vi "计算结果到报表.vi"(0 "步响应计算参数":T1, 1 "计算参数":T2, 2 "试验模式":string, 3 "试验报表路径":path) -> ()   [LabVIEW 2013]
doc: "该函数将计算所得的参数写入到试验报表的文本文档里。"
uses:
  <vilib>/Utility/config.llb/Write Key (String).vi
  <vilib>/Utility/config.llb/Write Key (Double).vi
  <vilib>/Utility/config.llb/NI_LVConfig.lvlib
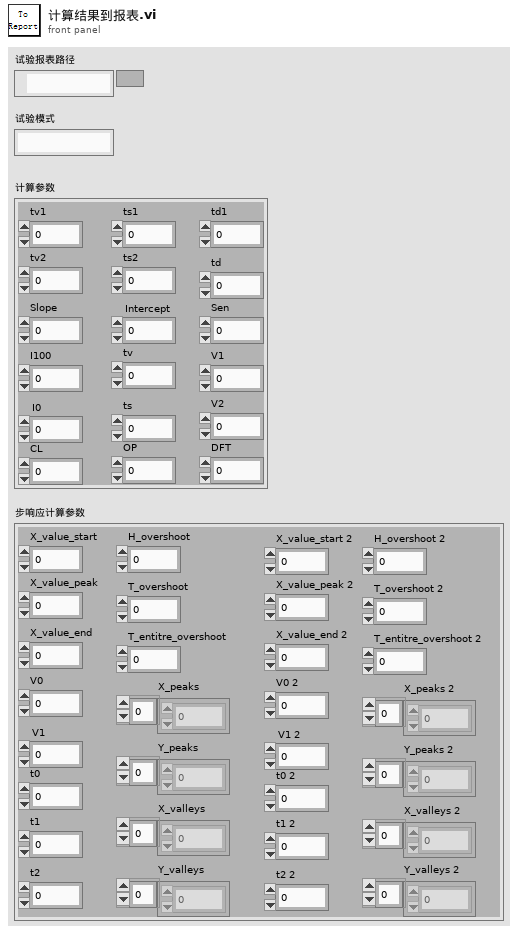
[diagram p1: front panel]
types:
  T1 = cluster{"X_value_start":dbl, "X_value_peak":dbl, "t1":dbl, "X_value_end":dbl, "V0":dbl, "V1":dbl, "t0":dbl, "X_peaks":dbl[], "X_valleys":dbl[], "Y_peaks":dbl[], "Y_valleys":dbl[], "t2":dbl, "H_overshoot":dbl, "T_overshoot":dbl, "T_entitre_overshoot":dbl, "X_value_start 2":dbl, "X_value_peak 2":dbl, "t1 2":dbl, "X_value_end 2":dbl, "V0 2":dbl, "V1 2":dbl, "t0 2":dbl, "X_peaks 2":dbl[], "X_valleys 2":dbl[], "Y_peaks 2":dbl[], "t2 2":dbl, "H_overshoot 2":dbl, "T_overshoot 2":dbl, "T_entitre_overshoot 2":dbl, "Y_valleys 2":dbl[]}
  T2 = cluster{"tv1":dbl, "tv2":dbl, "tv":dbl, "ts1":dbl, "ts2":dbl, "ts":dbl, "td1":dbl, "td":dbl, "Slope":dbl, "Intercept":dbl, "I100":dbl, "I0":dbl, "Sen":dbl, "V1":dbl, "V2":dbl, "CL":dbl, "OP":dbl, "DFT":dbl}
  T3 = typedef "NI_LVConfig.lvlib/Config Data RefNum.ctl" = refnum<k1>
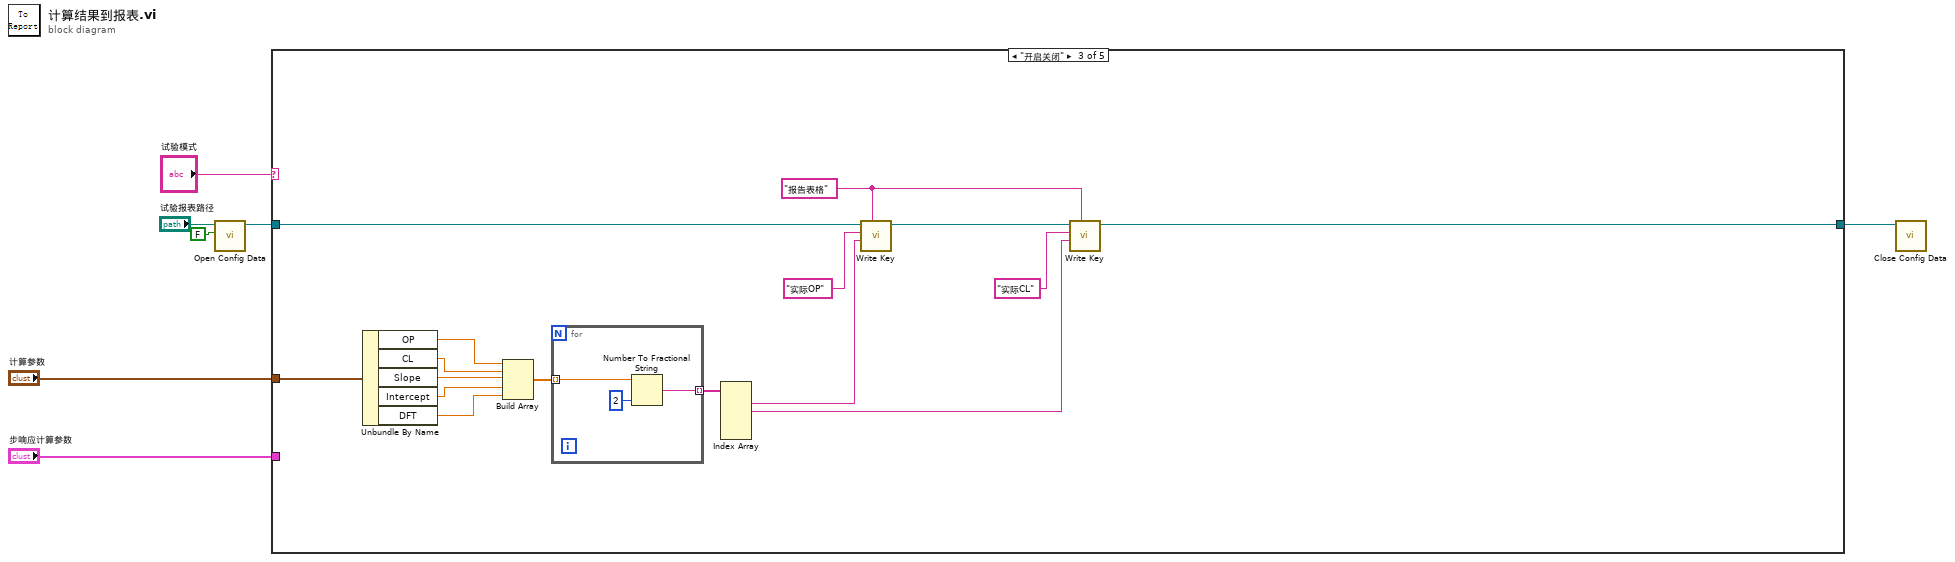
[diagram p0: block diagram]
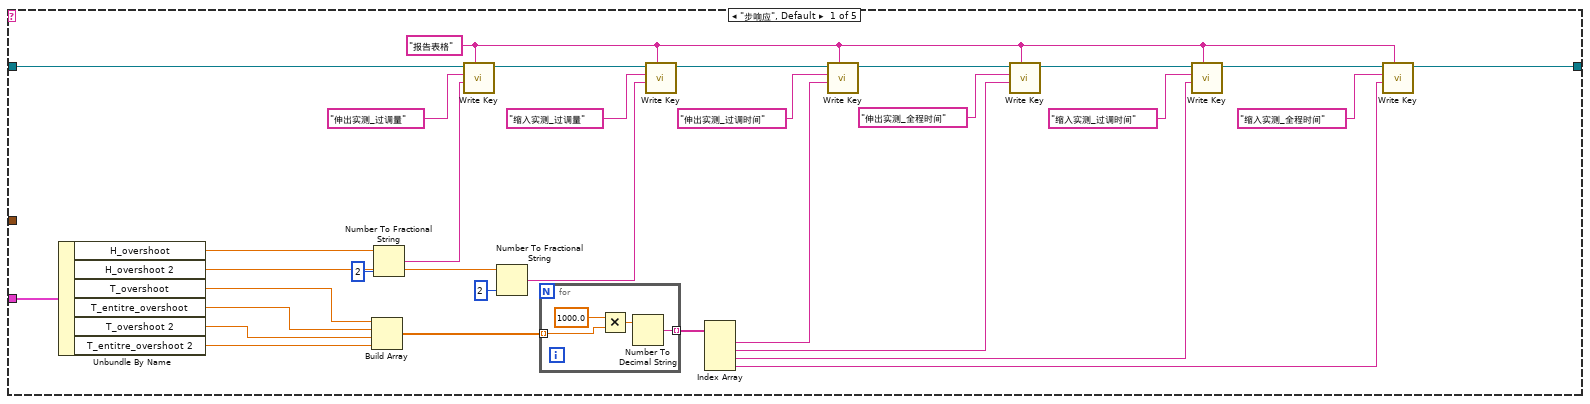
[diagram p2: hidden frame]
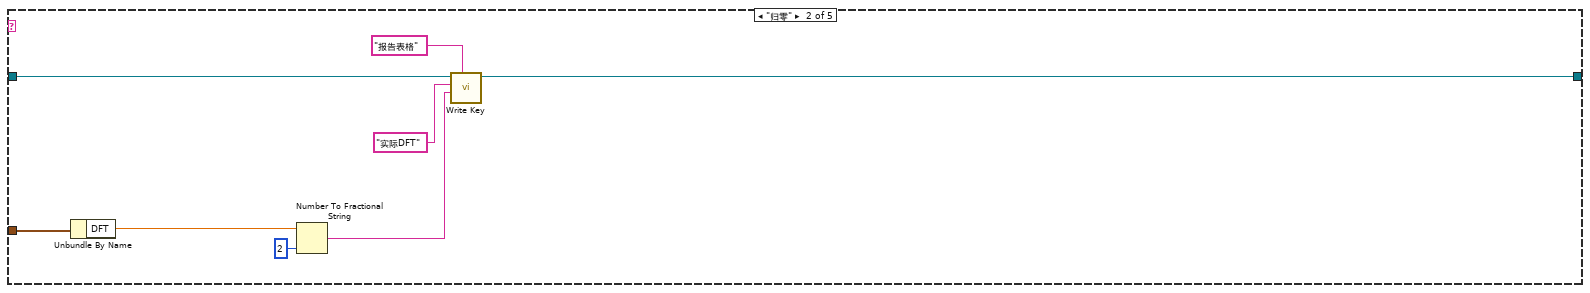
[diagram p3: hidden frame]
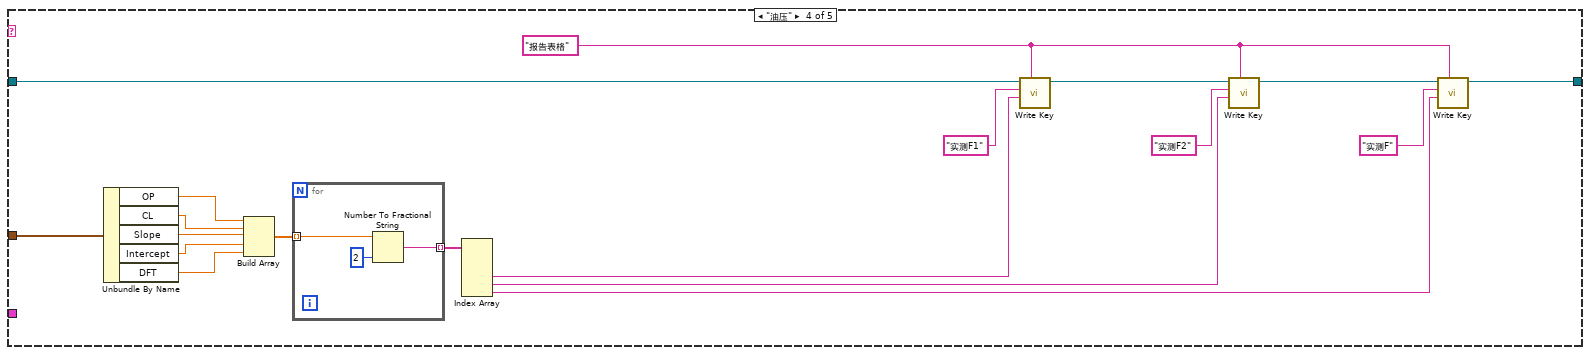
[diagram p4: hidden frame]
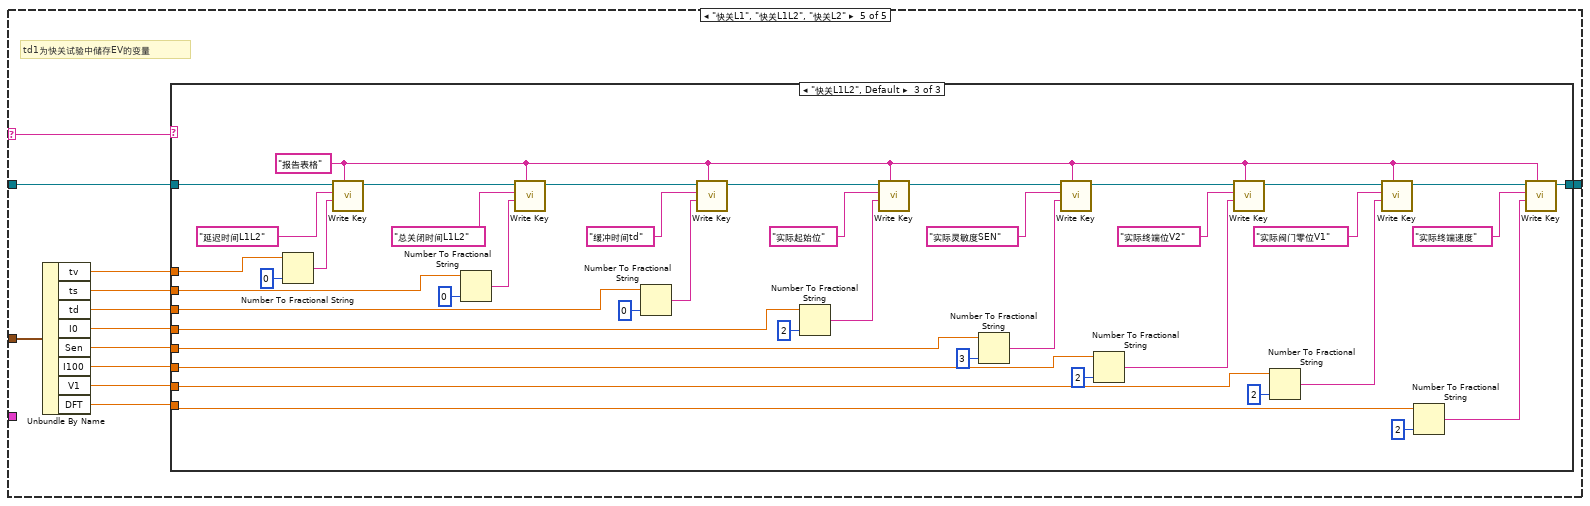
[diagram p5: hidden frame]
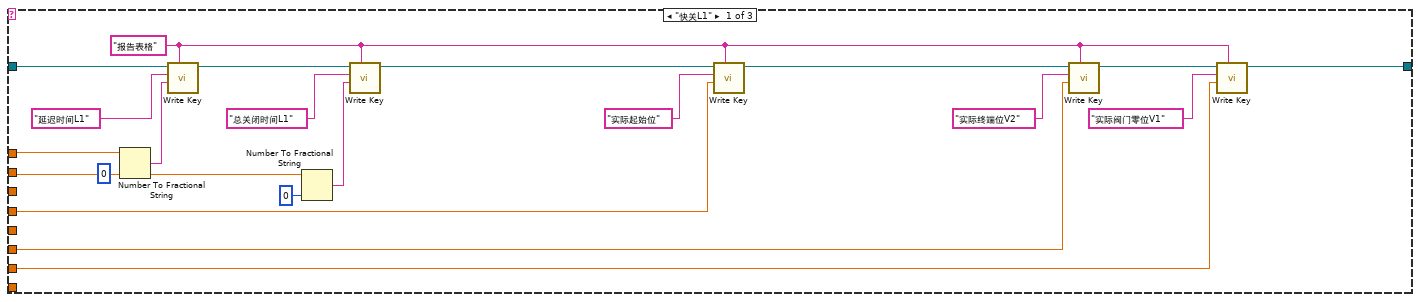
[diagram p6: hidden frame]
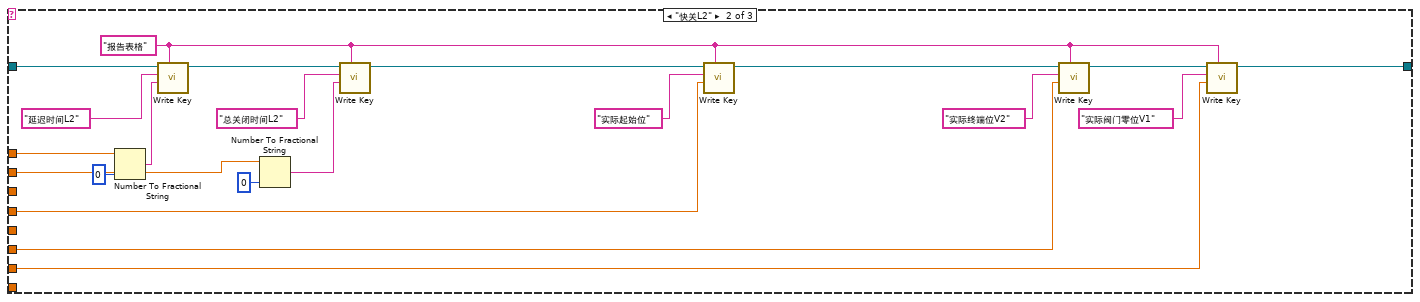
[diagram p7: hidden frame]
diagram:
  n1 = call <vilib>:"Open Config Data.vi"("create file if necessary (T)"=FALSE, "configuration file path"="试验报表路径") -> ("refnum"=w4:T3)  [unwired: 7 in, 2 out]
  n2 = case shown="\"开启关闭\"" "试验模式" {
    selector: "试验模式" -> [_ _ _ _ w103]
    tunnel: "计算参数" -> [_ w50 w66 w71 w102]
    tunnel: w4 -> [w29 w47 w62 w70 w101]
    tunnel: [w24 w46 w51 w72 w100] -> w3
    tunnel: "步响应计算参数" -> [w28 _ _ _ _]
    frame "步响应", Default {
      w26 = "报告表格"
      n3 = Unbundle By Name(w28) -> ("H_overshoot"=w12:dbl, "H_overshoot 2"=w9:dbl, "T_overshoot"=w20:dbl, "T_entitre_overshoot"=w21:dbl, "T_overshoot 2"=w18:dbl, "T_entitre_overshoot 2"=w22:dbl)
      n4 = Build Array(w20, w21, w18, w22) -> (w23:dbl[])
      n5 = Number To Fractional String(number=w12, precision (6)=i16 2) -> (F-format string=w11:string)  [unwired: 2 in]
      n6 = call-poly <vilib>:"Write Key.vi"("section"=w26, "value"=w11, "key"="伸出实测_过调量", "refnum"=w29) -> ("refnum out"=w33:T3)  [unwired: 5 in, 2 out]
      n7 = Number To Fractional String(number=w9, precision (6)=i16 2) -> (F-format string=w8:string)  [unwired: 2 in]
      n8 = for {
        tunnel: w23 -> [w41] mode=indexing
        tunnel: [w39] -> w19 mode=indexing
        n9 = Multiply(x=1000.0, y=w41) -> (x*y=w40:dbl)
        n10 = Number To Decimal String(number=w40) -> (decimal integer string=w39:string)  [unwired: 1 in]
      }
      n11 = call-poly <vilib>:"Write Key.vi"("section"=w26, "value"=w8, "key"="缩入实测_过调量", "refnum"=w33) -> ("refnum out"=w32:T3)  [unwired: 5 in, 2 out]
      n12 = Index Array(array=w19) -> (element #1=w17:string, element #2=w16:string, element #3=w15:string, element #4=w14:string)  [unwired: 4 in]
      n13 = call-poly <vilib>:"Write Key.vi"("section"=w26, "value"=w17, "key"="伸出实测_过调时间", "refnum"=w32) -> ("refnum out"=w31:T3)  [unwired: 5 in, 2 out]
      n14 = call-poly <vilib>:"Write Key.vi"("section"=w26, "value"=w16, "key"="伸出实测_全程时间", "refnum"=w31) -> ("refnum out"=w30:T3)  [unwired: 5 in, 2 out]
      n15 = call-poly <vilib>:"Write Key.vi"("section"=w26, "value"=w15, "key"="缩入实测_过调时间", "refnum"=w30) -> ("refnum out"=w25:T3)  [unwired: 5 in, 2 out]
      n16 = call-poly <vilib>:"Write Key.vi"("section"=w26, "value"=w14, "key"="缩入实测_全程时间", "refnum"=w25) -> ("refnum out"=w24:T3)  [unwired: 5 in, 2 out]
    }
    frame "归零" {
      n17 = Unbundle By Name(w50) -> ("DFT"=w45:dbl)
      n18 = Number To Fractional String(number=w45, precision (6)=i16 2) -> (F-format string=w44:string)  [unwired: 2 in]
      n19 = call-poly <vilib>:"Write Key.vi"("section"="报告表格", "value"=w44, "key"="实际DFT", "refnum"=w47) -> ("refnum out"=w46:T3)  [unwired: 5 in, 2 out]
    }
    frame "开启关闭" {
      w61 = "报告表格"
      n20 = Unbundle By Name(w66) -> ("OP"=w60:dbl, "CL"=w59:dbl, "Slope"=w58:dbl, "Intercept"=w57:dbl, "DFT"=w56:dbl)
      n21 = Build Array(w60, w59, w58, w57, w56) -> (w55:dbl[])
      n22 = for {
        tunnel: w55 -> [w68] mode=indexing
        tunnel: [w67] -> w54 mode=indexing
        n23 = Number To Fractional String(number=w68, precision (6)=i16 2) -> (F-format string=w67:string)  [unwired: 2 in]
      }
      n24 = Index Array(array=w54) -> (element #1=w53:string, element #2=w52:string)  [unwired: 5 in, 3 out]
      n25 = call-poly <vilib>:"Write Key.vi"("section"=w61, "value"=w53, "key"="实际OP", "refnum"=w62) -> ("refnum out"=w63:T3)  [unwired: 5 in, 2 out]
      n26 = call-poly <vilib>:"Write Key.vi"("section"=w61, "value"=w52, "key"="实际CL", "refnum"=w63) -> ("refnum out"=w51:T3)  [unwired: 5 in, 2 out]
    }
    frame "油压" {
      w78 = "报告表格"
      n27 = Unbundle By Name(w71) -> ("OP"=w79:dbl, "CL"=w80:dbl, "Slope"=w81:dbl, "Intercept"=w82:dbl, "DFT"=w83:dbl)
      n28 = Build Array(w79, w80, w81, w82, w83) -> (w84:dbl[])
      n29 = for {
        tunnel: w84 -> [w90] mode=indexing
        tunnel: [w89] -> w85 mode=indexing
        n30 = Number To Fractional String(number=w90, precision (6)=i16 2) -> (F-format string=w89:string)  [unwired: 2 in]
      }
      n31 = Index Array(array=w85) -> (element #3=w86:string, element #4=w87:string, element #5=w88:string)  [unwired: 5 in, 2 out]
      n32 = call-poly <vilib>:"Write Key.vi"("section"=w78, "value"=w86, "key"="实测F1", "refnum"=w70) -> ("refnum out"=w76:T3)  [unwired: 5 in, 2 out]
      n33 = call-poly <vilib>:"Write Key.vi"("section"=w78, "value"=w87, "key"="实测F2", "refnum"=w76) -> ("refnum out"=w77:T3)  [unwired: 5 in, 2 out]
      n34 = call-poly <vilib>:"Write Key.vi"("section"=w78, "value"=w88, "key"="实测F", "refnum"=w77) -> ("refnum out"=w72:T3)  [unwired: 5 in, 2 out]
    }
    frame "快关L1", "快关L1L2", "快关L2" {
      # "td1为快关试验中储存EV的变量"
      n35 = Unbundle By Name(w102) -> ("tv"=w99:dbl, "ts"=w98:dbl, "td"=w97:dbl, "I0"=w92:dbl, "Sen"=w93:dbl, "I100"=w94:dbl, "V1"=w95:dbl, "DFT"=w96:dbl)
      n36 = case shown="\"快关L1L2\", Default" w103 {
        tunnel: w101 -> [w116 w145 w171]
        tunnel: [w105 w127 w170] -> w100
        tunnel: w99 -> [w107 w128 w149]
        tunnel: w98 -> [w110 w131 w152]
        tunnel: w97 -> [_ _ w155]
        tunnel: w92 -> [w113 w139 w146]
        tunnel: w93 -> [_ _ w167]
        tunnel: w94 -> [w114 w138 w164]
        tunnel: w95 -> [w115 w137 w161]
        tunnel: w96 -> [_ _ w158]
        frame "快关L1" {
          w117 = "报告表格"
          n37 = Number To Fractional String(number=w107, precision (6)=i16 0) -> (F-format string=w108:string)  [unwired: 2 in]
          n38 = call-poly <vilib>:"Write Key.vi"("section"=w117, "value"=w108, "key"="延迟时间L1", "refnum"=w116) -> ("refnum out"=w119:T3)  [unwired: 5 in, 2 out]
          n39 = Number To Fractional String(number=w110, precision (6)=i16 0) -> (F-format string=w111:string)  [unwired: 2 in]
          n40 = call-poly <vilib>:"Write Key.vi"("section"=w117, "value"=w111, "key"="总关闭时间L1", "refnum"=w119) -> ("refnum out"=w106:T3)  [unwired: 5 in, 2 out]
          n41 = call-poly <vilib>:"Write Key.vi"("section"=w117, "value"=w113, "key"="实际起始位", "refnum"=w106) -> ("refnum out"=w104:T3)  [unwired: 5 in, 2 out]
          n42 = call-poly <vilib>:"Write Key.vi"("section"=w117, "value"=w114, "key"="实际终端位V2", "refnum"=w104) -> ("refnum out"=w118:T3)  [unwired: 5 in, 2 out]
          n43 = call-poly <vilib>:"Write Key.vi"("section"=w117, "value"=w115, "key"="实际阀门零位V1", "refnum"=w118) -> ("refnum out"=w105:T3)  [unwired: 5 in, 2 out]
        }
        frame "快关L2" {
          w134 = "报告表格"
          n44 = Number To Fractional String(number=w128, precision (6)=i16 0) -> (F-format string=w129:string)  [unwired: 2 in]
          n45 = call-poly <vilib>:"Write Key.vi"("section"=w134, "value"=w129, "key"="延迟时间L2", "refnum"=w145) -> ("refnum out"=w136:T3)  [unwired: 5 in, 2 out]
          n46 = Number To Fractional String(number=w131, precision (6)=i16 0) -> (F-format string=w132:string)  [unwired: 2 in]
          n47 = call-poly <vilib>:"Write Key.vi"("section"=w134, "value"=w132, "key"="总关闭时间L2", "refnum"=w136) -> ("refnum out"=w126:T3)  [unwired: 5 in, 2 out]
          n48 = call-poly <vilib>:"Write Key.vi"("section"=w134, "value"=w139, "key"="实际起始位", "refnum"=w126) -> ("refnum out"=w125:T3)  [unwired: 5 in, 2 out]
          n49 = call-poly <vilib>:"Write Key.vi"("section"=w134, "value"=w138, "key"="实际终端位V2", "refnum"=w125) -> ("refnum out"=w135:T3)  [unwired: 5 in, 2 out]
          n50 = call-poly <vilib>:"Write Key.vi"("section"=w134, "value"=w137, "key"="实际阀门零位V1", "refnum"=w135) -> ("refnum out"=w127:T3)  [unwired: 5 in, 2 out]
        }
        frame "快关L1L2", Default {
          w172 = "报告表格"
          n51 = Number To Fractional String(number=w149, precision (6)=i16 0) -> (F-format string=w150:string)  [unwired: 2 in]
          n52 = call-poly <vilib>:"Write Key.vi"("section"=w172, "value"=w150, "key"="延迟时间L1L2", "refnum"=w171) -> ("refnum out"=w179:T3)  [unwired: 5 in, 2 out]
          n53 = Number To Fractional String(number=w152, precision (6)=i16 0) -> (F-format string=w153:string)  [unwired: 2 in]
          n54 = call-poly <vilib>:"Write Key.vi"("section"=w172, "value"=w153, "key"="总关闭时间L1L2", "refnum"=w179) -> ("refnum out"=w178:T3)  [unwired: 5 in, 2 out]
          n55 = Number To Fractional String(number=w155, precision (6)=i16 0) -> (F-format string=w156:string)  [unwired: 2 in]
          n56 = call-poly <vilib>:"Write Key.vi"("section"=w172, "value"=w156, "key"="缓冲时间td", "refnum"=w178) -> ("refnum out"=w177:T3)  [unwired: 5 in, 2 out]
          n57 = Number To Fractional String(number=w146, precision (6)=i16 2) -> (F-format string=w147:string)  [unwired: 2 in]
          n58 = call-poly <vilib>:"Write Key.vi"("section"=w172, "value"=w147, "key"="实际起始位", "refnum"=w177) -> ("refnum out"=w176:T3)  [unwired: 5 in, 2 out]
          n59 = Number To Fractional String(number=w167, precision (6)=i16 3) -> (F-format string=w168:string)  [unwired: 2 in]
          n60 = call-poly <vilib>:"Write Key.vi"("section"=w172, "value"=w168, "key"="实际灵敏度SEN", "refnum"=w176) -> ("refnum out"=w175:T3)  [unwired: 5 in, 2 out]
          n61 = Number To Fractional String(number=w164, precision (6)=i16 2) -> (F-format string=w165:string)  [unwired: 2 in]
          n62 = call-poly <vilib>:"Write Key.vi"("section"=w172, "value"=w165, "key"="实际终端位V2", "refnum"=w175) -> ("refnum out"=w174:T3)  [unwired: 5 in, 2 out]
          n63 = Number To Fractional String(number=w161, precision (6)=i16 2) -> (F-format string=w162:string)  [unwired: 2 in]
          n64 = call-poly <vilib>:"Write Key.vi"("section"=w172, "value"=w162, "key"="实际阀门零位V1", "refnum"=w174) -> ("refnum out"=w173:T3)  [unwired: 5 in, 2 out]
          n65 = Number To Fractional String(number=w158, precision (6)=i16 2) -> (F-format string=w159:string)  [unwired: 2 in]
          n66 = call-poly <vilib>:"Write Key.vi"("section"=w172, "value"=w159, "key"="实际终端速度", "refnum"=w173) -> ("refnum out"=w170:T3)  [unwired: 5 in, 2 out]
        }
      }
    }
  }
  n67 = call <vilib>:"Close Config Data.vi"("refnum"=w3) -> ()  [unwired: 9 in, 2 out]
